vi "RunTests.vi"() -> (2 "successful?":bool, 3 "test details":string)   [LabVIEW 2018]
uses:
  CarWashTestSuite/CarWashTestSuite.lvclass
  C:/Program Files/National Instruments/LabVIEW 2018/vi.lib/addons/_JKI Toolkits/VI Tester/TestSuite.llb/TestSuite.lvclass
  <vilib>/addons/_JKI Toolkits/VI Tester/VI Tester API.llb/Run Tests (TestSuite Object).vi
  <vilib>/addons/_JKI Toolkits/VI Tester/VI Tester API.llb/VI Tester API.lvlib
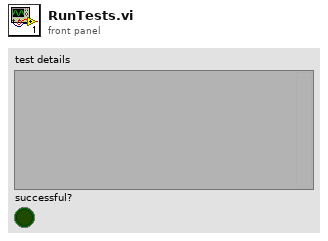
[diagram p1: front panel]
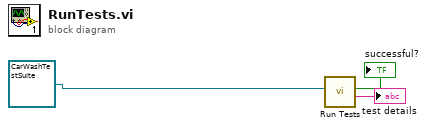
[diagram p0: block diagram]
diagram:
  n1 = call-poly <vilib>:"Run Tests.vi"("TestSuite"=refnum<class "CarWashTestSuite.lvclass"> refnum ("CarWashTestSuite.lvclass")) -> ("test details"=→"test details":string, "successful?"=→"successful?":bool)  [unwired: 8 in, 1 out]
